vi "S2C_PCIe7841_Proc_Initialize.vi"(8 "Error In":errorcluster) -> (0 "Error Out":errorcluster)   [LabVIEW 2015]
uses:
  S2C_PCIe7841_Proc_Globals.vi
  <vilib>/rvi/interface/RandomDataEmulation/nirviRandomDataOpen.vi
  <vilib>/rvi/interface/common/niFpgaCacheSessionInfoDynamic.vi
  <vilib>/rvi/interface/nirviOpenFPGA/nirviOpenFPGA.xnode
  FPGA/S2C_FPGA_Main.vi
  Builds/S2C_PCIe7841/S2CProject_FPGATarget_(Bit-Level).lvbitx
  <vilib>/FPGAPlugInAG/PCIe-7841R/niLvFpga_Open_PCIe-7841R.vi
  <vilib>/rvi/interface/common/dynamic/niFpgaDynamicAddResources.vi
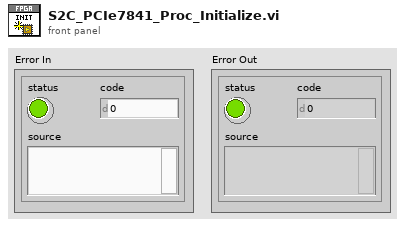
[diagram p1: front panel]
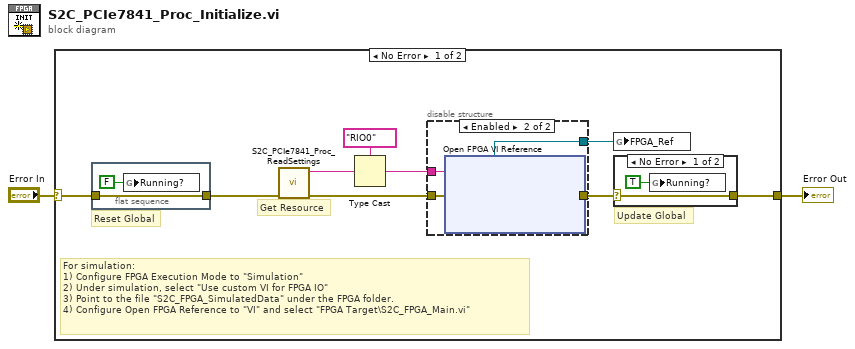
[diagram p0: block diagram]
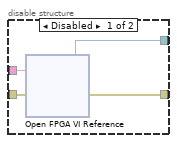
[diagram p2: hidden frame]
diagram:
  n1 = case shown="No Error" "Error In" {
    selector: "Error In" -> [w11 w25]
    tunnel: [w9 w25] -> w1
    frame No Error {
      # "Get Resource"
      # "For simulation:\n1) Configure FPGA Execution Mode to \"Simulation\"\n2) Under simulation, select \"Use custom VI for FPGA IO\"\n3) Point to the file \"S2C_FPGA_SimulatedData\" under the FPGA folder.\n4) Configure Open FPGA Reference to \"VI\" and select \"FPGA Target\\S2C_FPGA_Main.vi\""
      # "Update Global"
      # "Reset Global"
      n2 = flat-sequence {
        tunnel: w11 -> [w23]
        tunnel: [w23] -> w5
        frame #0 {
          n3 = global write "S2C_PCIe7841_Proc_Globals.vi" "Running?"(FALSE ("Running?")) -> ()
        }
      }
      n4 = call "S2C_PCIe7841_Proc_ReadSettings.vi"("Error In"=w5) -> ("Error Out"=w4:errorcluster, "ResourceName"=w3:string)  [unwired: 9 in]
      n5 = Type Cast(type=tag "RIO0" ("resource name"), x=w3) -> (*(type *) &x=w6:tag)
      n6 = disable-structure shown="Enabled" {
        disable-tunnel: w4 -> [w15 w19]
        disable-tunnel: [w14 w18] -> w10
        disable-tunnel: [w13 w17] -> w8
        disable-tunnel: w6 -> [w12 w16]
        frame Disabled {
          n7 = xnode "Open FPGA VI Reference"("error in"=w15, "resource name"=w12) -> ("FPGA VI Reference Out"=w13:refnum<k20>, "error out"=w14:errorcluster)
        }
        frame Enabled {
          n8 = xnode "Open FPGA VI Reference"("error in"=w19, "resource name"=w16) -> ("FPGA VI Reference Out"=w17:refnum<k20>, "error out"=w18:errorcluster)
        }
      }
      n9 = global write "S2C_PCIe7841_Proc_Globals.vi" "FPGA_Ref"(w8) -> ()
      n10 = case shown="No Error" w10 {
        selector: w10 -> [w21 w22]
        tunnel: [w21 w22] -> w9
        frame No Error {
          n11 = global write "S2C_PCIe7841_Proc_Globals.vi" "Running?"(TRUE ("Running?")) -> ()
        }
        frame Error {
        }
      }
    }
    frame Error {
    }
  }
  "Error Out" <- w1
